vi "Init.vi"(8 "error in":errorcluster, 11 "PCAN in":refnum<class "PCAN.lvclass">) -> (0 "error out":errorcluster, 3 "PCAN out":refnum<class "PCAN.lvclass">)   [LabVIEW 2023, in "PCAN.lvclass"]
uses:
  PCAN.lvclass
  PCAN.lvclass/PCAN.ctl
  <instrlib>/KDI Digital Instrumentation/API_for_PCAN_BASIC_FD/TPCANHandle.ctl
  <instrlib>/KDI Digital Instrumentation/API_for_PCAN_BASIC_FD/TPCANParameter.ctl
  Configuration/Configuration JSON/Configuration JSON Base/CFG JSON.lvclass
  <instrlib>/KDI Digital Instrumentation/API_for_PCAN_BASIC_FD/TPCANBaudrate.ctl
  D:/git/HAL/HAL GOOP4/Configuration/Configuration JSON/Configuration JSON Base/CFG JSON.lvclass
  D:/git/HAL/HAL GOOP4/Interfaces/IConfigure/IConfigure.lvclass
  D:/git/HAL/HAL GOOP4/Devices/CAN Interfaces/PCAN/PCAN.lvclass
  D:/git/HAL/HAL GOOP4/Protocols/ICAN/ICAN.lvclass
  c7398602-ee2b-4d62-8e4d-34dfde18aa1c.vi
  <instrlib>/KDI Digital Instrumentation/API_for_PCAN_BASIC_FD/Error language selector.ctl
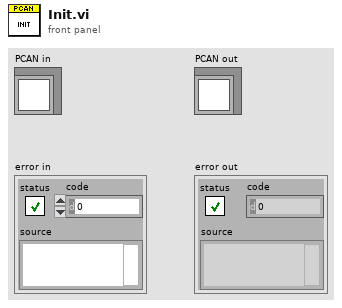
[diagram p1: front panel]
types:
  T1 = typedef "TPCANBaudrate.ctl" = enum16{"PCAN_BAUD_1M 0x0014", "PCAN_BAUD_800K 0x0016", "PCAN_BAUD_500K 0x001C", "PCAN_BAUD_250K 0x011C", "PCAN_BAUD_125K 0x031C", "PCAN_BAUD_100K 0x432F", "PCAN_BAUD_95K 0xC34E", "PCAN_BAUD_83K 0x852B", "PCAN_BAUD_50K 0x472F", "PCAN_BAUD_47K 0x1414", "PCAN_BAUD_33K 0x8B2F", "PCAN_BAUD_20K 0x532F", "PCAN_BAUD_10K 0x672F", "PCAN_BAUD_5K 0x7F7F", "User Baudrate"}
  T2 = typedef "TPCANHandle.ctl" = enum16{"PCAN_NONEBUS  0x000", "PCAN_ISABUS1  0x21", "PCAN_ISABUS2  0x22", "PCAN_ISABUS3  0x23", "PCAN_ISABUS4  0x24", "PCAN_ISABUS5  0x25", "PCAN_ISABUS6  0x26", "PCAN_ISABUS7  0x27", "PCAN_ISABUS8  0x28", "PCAN_DNGBUS1  0x31", "PCAN_PCIBUS1  0x41", "PCAN_PCIBUS1  0x42", "PCAN_PCIBUS1  0x43", "PCAN_PCIBUS1  0x44", "PCAN_PCIBUS1  0x45", "PCAN_PCIBUS1  0x46", "PCAN_PCIBUS1  0x47", "PCAN_PCIBUS1  0x48", "PCAN_PCIBUS1  0x409", "PCAN_PCIBUS1  0x40A", "PCAN_PCIBUS1  0x40B", "PCAN_PCIBUS1  0x40C", "PCAN_PCIBUS1  0x40D", "PCAN_PCIBUS1  0x40E", "PCAN_PCIBUS1  0x40F", "PCAN_PCIBUS1  0x410", "PCAN_USBBUS1  0x51", "PCAN_USBBUS2  0x52", "PCAN_USBBUS3  0x53", "PCAN_USBBUS4  0x54", "PCAN_USBBUS5  0x55", "PCAN_USBBUS6  0x56", "PCAN_USBBUS7  0x57", "PCAN_USBBUS8  0x58", "PCAN_USBBUS9  0x509", "PCAN_USBBUS10  0x50A", "PCAN_USBBUS11  0x50B", "PCAN_USBBUS12  0x50C", "PCAN_USBBUS13  0x50D", "PCAN_USBBUS14  0x50E", "PCAN_USBBUS15  0x50F", "PCAN_USBBUS16  0x510", "PCAN_PCCBUS1  0x61", "PCAN_PCCBUS2  0x62", "PCAN_LANBUS1  0x801", "PCAN_LANBUS2  0x802", "PCAN_LANBUS3  0x803", "PCAN_LANBUS4  0x804", "PCAN_LANBUS5  0x805", "PCAN_LANBUS6  0x806", "PCAN_LANBUS7  0x807", "PCAN_LANBUS8  0x808", "PCAN_LANBUS9  0x809", "PCAN_LANBUS10  0x80A", "PCAN_LANBUS11  0x80B", "PCAN_LANBUS12  0x80C", "PCAN_LANBUS13  0x80D", "PCAN_LANBUS14  0x80E", "PCAN_LANBUS15  0x80F", "PCAN_LANBUS16  0x810"}
  T3 = typedef "TPCANParameter.ctl" = enum8{"Not Available", "PCAN device number", "PCAN 5-volt power", "PCAN receive event", "PCAN message filter", "PCAN API version", "PCAN channel version", "PCAN busoff autoreset", "PCAN listen-only", "PCAN log location", "PCAN log status", "PCAN log configure", "PCAN log text", "PCAN channel condition", "PCAN hardware name", "PCAN_RECEIVE_STATUS", "PCAN_CONTROLLER_NUMBER", "PCAN_TRACE_LOCATION ", "PCAN_TRACE_STATUS", "PCAN_TRACE_SIZE", "PCAN_TRACE_CONFIGURE", "PCAN_CHANNEL_IDENTIFYING", "PCAN_CHANNEL_FEATURES", "PCAN_SPEED_ADAPTING", "PCAN_BITRATE_INFO", "PCAN_BITRATE_INFO_FD", "PCAN_BUSSPEED_NOMINAL", "PCAN_BUSSPEED_DATA", "PCAN_IP_ADDRESS", "PCAN_LAN_SERVICE_STATUS", "PCAN_ALLOW_STATUS_FRAMES", "PCAN_ALLOW_RTR_FRAMES", "PCAN_ALLOW_ERROR_FRAMES", "PCAN_INTERFRAME_DELAY", "PCAN_ACCEPTANCE_FILTER_11BIT", "PCAN_ACCEPTANCE_FILTER_29BIT", "PCAN_IO_DIGITAL_CONFIGURATION", "PCAN_IO_DIGITAL_VALUE", "PCAN_IO_DIGITAL_SET", "PCAN_IO_DIGITAL_CLEAR", "PCAN_IO_ANALOG_VALUE", "PCAN_FIMRWARE_VRSION", "PCAN__ATTACHED_CHANNELS_COUNT", "PCAN_ATTACHED CHANNELS"}
  T4 = typedef "Error language selector.ctl" = u16
  T5 = typedef "Channel Availability.ctl" = enum16{"PCAN_CHANNEL_UNAVAILABLE", "PCAN_CHANNEL_AVAILABLE", "PCAN_CHANNEL_OCCUPIED", "PCAN_CHANNEL_PCANVIEW "}
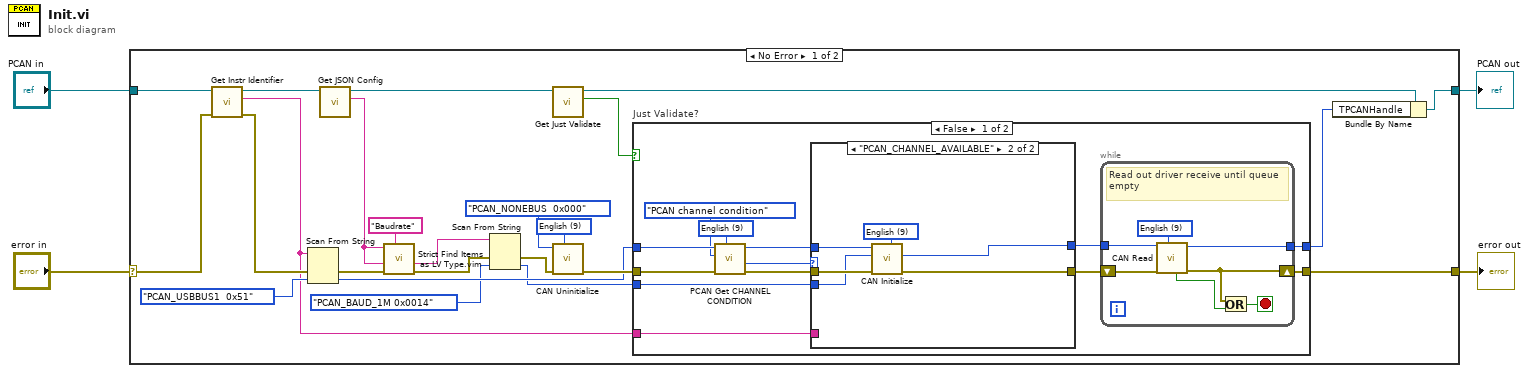
[diagram p0: block diagram]
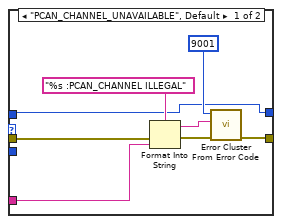
[diagram p2: hidden frame]
diagram:
  n1 = case shown="No Error" "error in" {
    selector: "error in" -> [w20 w66]
    tunnel: [w25 w66] -> w3
    tunnel: [w16 w65] -> w2
    tunnel: "PCAN in" -> [w22 w65]
    frame No Error {
      w5 = T4 9 items=["System dependent", "Not available", "Not available", "Not available", "Not available", "Not available", "Not available", "Deutsch", "Not available", "English", "Español", "Not available", "Français", "Not available", "Not available", "Not available", "Italiano"] ("Language")
      n2 = call-dynamic "Get Instr Identifier.vi"("error in"=w20, "Configuration Base in"=w22) -> ("error out"=w19:errorcluster, "Instr Ident"=w18:string, "Configuration Base out"=w21:refnum<class "PCAN.lvclass">)  [unwired: 7 in]
      n3 = Scan From String(input string=w18, error in=w19, default 1=TPCANHandle."PCAN_USBBUS1  0x51" ("TPCANHandle")) -> (error out=w26:errorcluster, output 1=w24:T2)  [unwired: 2 in, 2 out]
      n4 = call "Get JSON Config.vi"("CFG Base in"=w21) -> ("<JSON>Config>"=w10:string, "CFG Base out"=w12:refnum<class "PCAN.lvclass">)  [unwired: 9 in]
      n5 = call "Strict Find Items as LV Type.vim"("$Path or Item Name"="Baudrate", "error in"=w26, "Data Type and Default Value"=w10, "JSON"=w10) -> ("error out"=w11:errorcluster, "Data out"=w8:string)  [unwired: 6 in]
      n6 = Scan From String(input string=w8, error in=w11, default 1=TPCANBaudrate."PCAN_BAUD_1M 0x0014" ("TPCANBaudrate")) -> (error out=w13:errorcluster, output 1=w7:T1)  [unwired: 2 in, 2 out]
      n7 = call "Get Just Validate.vi"("CFG JSON Base in"=w12) -> ("Just Validate"=w14:bool, "CFG JSON Base out"=w17:refnum<class "PCAN.lvclass">)  [unwired: 9 in]
      n8 = call <instrlib>:"CAN Uninitialize.vi"("Language"=w5, "error in (no error)"=w13, "TPCANHandle"=TPCANHandle."PCAN_NONEBUS  0x000") -> ("error out"=w28:errorcluster)  [unwired: 6 in, 2 out]
      n9 = case "Just Validate?" shown="False" w14 {
        tunnel: w28 -> [w41 w64]
        tunnel: [w35 w64] -> w25
        tunnel: w24 -> [w34 w63]
        tunnel: w18 -> [w33 _]
        tunnel: [w32 w63] -> w15
        tunnel: w7 -> [w30 _]
        frame False {
          w29 = T4 9 items=["System dependent", "Not available", "Not available", "Not available", "Not available", "Not available", "Not available", "Deutsch", "Not available", "English", "Español", "Not available", "Français", "Not available", "Not available", "Not available", "Italiano"] ("Language")
          n10 = call <instrlib>:"PCAN Get CHANNEL CONDITION.vi"("Language"=w29, "error in (no error)"=w41, "TPCANParameter"=TPCANParameter."PCAN channel condition", "TPCANHandle"=w34) -> ("error out"=w40:errorcluster, "Channel condition"=w39:T5, "TPCANHandle out"=w38:T2)  [unwired: 5 in]
          n11 = case shown="\"PCAN_CHANNEL_AVAILABLE\"" w39 {
            tunnel: w40 -> [w53 w62]
            tunnel: [w56 w61] -> w37
            tunnel: w38 -> [w50 w60]
            tunnel: [w50 w59] -> w36
            tunnel: w33 -> [w49 _]
            tunnel: w30 -> [_ w58]
            frame "PCAN_CHANNEL_UNAVAILABLE", Default {
              n12 = Format Into String(format string="%s :PCAN_CHANNEL ILLEGAL" ("source"), error in=w53, w49) -> (resulting string=w51:string, error out=w52:errorcluster)  [unwired: 1 in]
              n13 = call <vilib>:"Error Cluster From Error Code.vi"("error in (no error)"=w52, "error message (\"\")"=w51, "error code (0)"=9001) -> ("error out"=w56:errorcluster)  [unwired: 6 in]
            }
            frame "PCAN_CHANNEL_AVAILABLE" {
              w57 = T4 9 items=["System dependent", "Not available", "Not available", "Not available", "Not available", "Not available", "Not available", "Deutsch", "Not available", "English", "Español", "Not available", "Français", "Not available", "Not available", "Not available", "Italiano"] ("Language")
              n14 = call <instrlib>:"CAN Initialize.vi"("Language"=w57, "error in (no error)"=w62, "TPCANBaudrate"=w58, "TPCANHandle"=w60) -> ("error out"=w61:errorcluster, "TPCANHandle_out"=w59:T2)  [unwired: 5 in, 1 out]
            }
          }
          n15 = while {
            shift-right: [w46] -> w35
            shift-left: w37 -> [w48]
            tunnel: w36 -> [w44]
            tunnel: [w43] -> w32
            stop <- w47 stop-if-true
            w42 = T4 9 items=["System dependent", "Not available", "Not available", "Not available", "Not available", "Not available", "Not available", "Deutsch", "Not available", "English", "Español", "Not available", "Français", "Not available", "Not available", "Not available", "Italiano"] ("Language")
            # "Read out driver receive until queue empty"
            n16 = call <instrlib>:"CAN Read.vi"("Language"=w42, "error in (no error)"=w48, "TPCANHandle"=w44) -> ("error out"=w46:errorcluster, "TPCANHandle out"=w43:T2, "rcv queue empty"=w45:bool)  [unwired: 4 in, 2 out]
            n17 = Or(x=w46, y=w45) -> (x .or. y?=w47:bool)
          }
        }
        frame True {
        }
      }
      n18 = Bundle By Name(cluster=w17, "TPCANHandle"=w15) -> (w16:refnum<class "PCAN.lvclass">)
    }
    frame Error {
    }
  }
  "error out" <- w3
  "PCAN out" <- w2
